vi "Stop.vi"(8 "error in (no error)":errorcluster, 11 "Stop Message in":refnum<class "Stop Message.lvclass">) -> (0 "error out":errorcluster, 3 "Stop Message out":refnum<class "Stop Message.lvclass">)   [LabVIEW 2010, in "Stop Message.lvclass"]
uses:
  Stop Message.lvclass
  Advanced Waveform Class/Advanced Waveform.lvclass
  Message.lvclass
panel:
  in  "Command queue":refnum<queue>
  out "Advanced Waveform Out":refnum<class "Advanced Waveform.lvclass">
  in  "Advanced Waveform In":refnum<class "Advanced Waveform.lvclass">
  out "Stop":bool
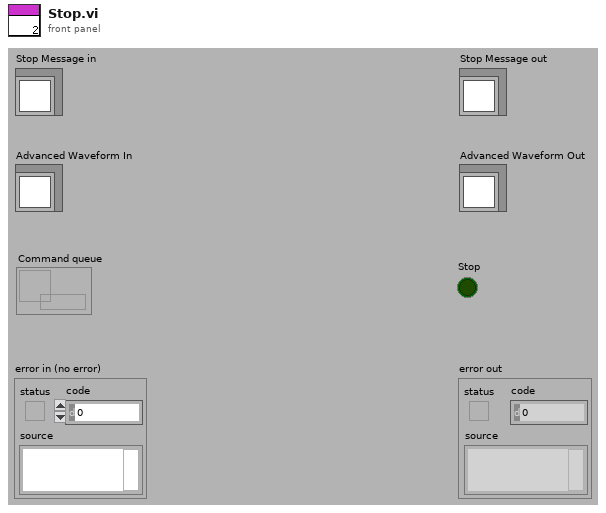
[diagram p1: front panel]
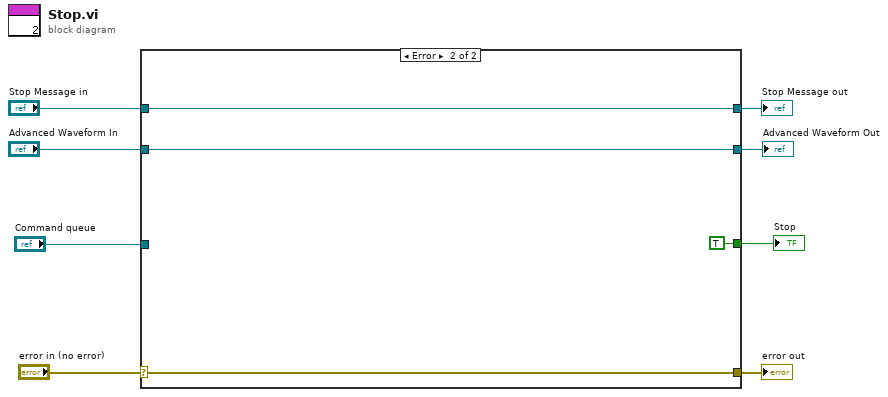
[diagram p0: block diagram]
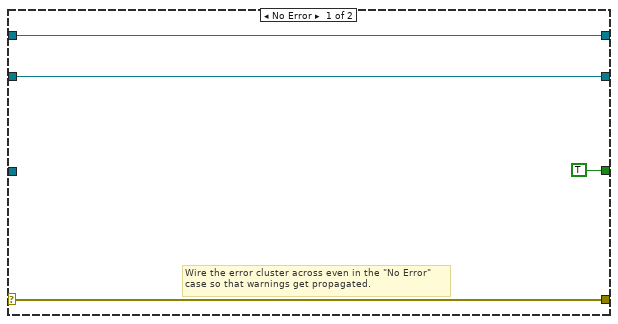
[diagram p2: hidden frame]
diagram:
  n1 = case shown="Error" "error in (no error)" {
    selector: "error in (no error)" -> [w11 w16]
    tunnel: [w11 w16] -> w7
    tunnel: [w12 w15] -> w5
    tunnel: "Stop Message in" -> [w12 w15]
    tunnel: "Advanced Waveform In" -> [w10 w14]
    tunnel: [w10 w14] -> w3
    tunnel: "Command queue" -> [_ _]
    tunnel: [TRUE TRUE] -> w1
    frame No Error {
      # "Wire the error cluster across even in the \"No Error\"\ncase so that warnings get propagated."
    }
    frame Error {
    }
  }
  "error out" <- w7
  "Stop Message out" <- w5
  "Advanced Waveform Out" <- w3
  "Stop" <- w1
